vi "Case Structures.vi"() -> ()   [LabVIEW 2014]
panel:
  out "随机值":dbl
  in  "错误输入（无错误）":cluster{"状态":bool, "代码":i32, "源":string}
  in  "枚举选择":enum16{"选项A", "选项B", "选项C"}(ring)
  in  "字符串选择":string
  in  "数值选择":i32
  in  "布尔选择":bool
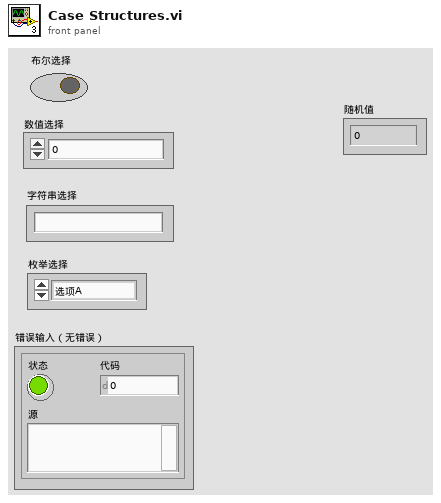
[diagram p1: front panel]
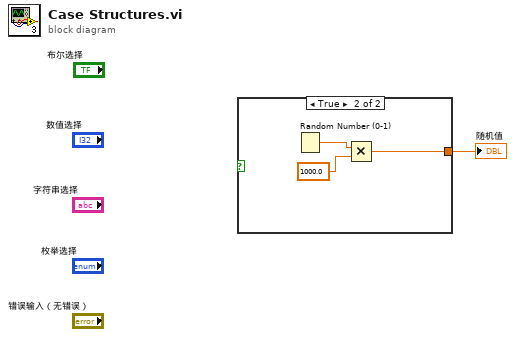
[diagram p0: block diagram]
diagram:
  n1 = case shown="True" {
    selector: _ -> [_ _]
    tunnel: [_ w2] -> w1
    frame False {
    }
    frame True {
      n2 = Random Number (0-1)() -> (number: 0 to 1=w4:dbl)
      n3 = Multiply(x=w4, y=1000.0) -> (x*y=w2:dbl)
    }
  }
  "随机值" <- w1
